vi "Get Memory Size.vi"(8 "error in(no error)":errorcluster, 11 "VISA Resource Name":refnum<visa-resource-name>) -> (0 "error out":errorcluster, 1 "subprog memory [B]":i32, 2 "sample memory [B]":i32, 3 "VISA resource name out":refnum<visa-resource-name>)   [LabVIEW 2020, in "3458A Basic Driver.lvlib"]
doc: "Reads memory size of the 3458A unit. Both memory sizez are in bytes."
uses:
  3458A Basic Driver.lvlib
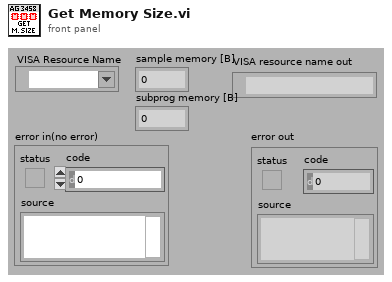
[diagram p1: front panel]
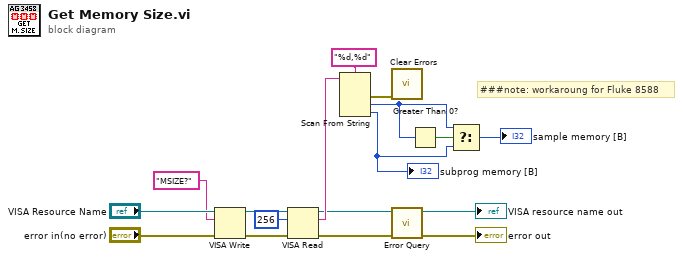
[diagram p0: block diagram]
diagram:
  # "###note: workaroung for Fluke 8588"
  n1 = VISA Write(VISA resource name="VISA Resource Name", write buffer="MSIZE?", error in (no error)="error in(no error)") -> (VISA resource name out=w13:refnum<visa-resource-name>, error out=w14:errorcluster)  [unwired: 1 out]
  n2 = VISA Read(VISA resource name=w13, byte count=u32 256, error in (no error)=w14) -> (VISA resource name out=w7:refnum<visa-resource-name>, read buffer=w8:string, error out=w9:errorcluster)  [unwired: 1 out]
  n3 = Scan From String(format string="%d,%d", input string=w8) -> (error out=w10:errorcluster, output 1=w3:i32, output 2=w2:i32)  [unwired: 4 in, 2 out]
  "subprog memory [B]" <- w2
  n4 = call <vilib>:"Clear Errors.vi"("error in (no error)"=w10) -> ()  [unwired: 5 in, 2 out]
  n5 = call "Error Query.vi"("error in (no error)"=w9, "VISA resource name"=w7) -> ("error out"=→"error out":errorcluster, "VISA resource name out"=→"VISA resource name out":refnum<visa-resource-name>)  [unwired: 6 in, 2 out]
  n6 = Greater Than 0?(x=w3) -> (x > 0?=w4:bool)
  n7 = Select(t=w3, s=w4, f=w2) -> (s? t:f=→"sample memory [B]":i32)
